vi "generic_PID.vi"(6 "initiation":dbl format="%#_13g", 7 "sensor input":dbl, 8 "setpoint":dbl, 9 "Kd":dbl format="%#_13g", 10 "KI":dbl format="%#_13g", 11 "Kp":dbl format="%#_13g") -> (1 "error":dbl, 2 "PID":dbl)   [LabVIEW 2018]
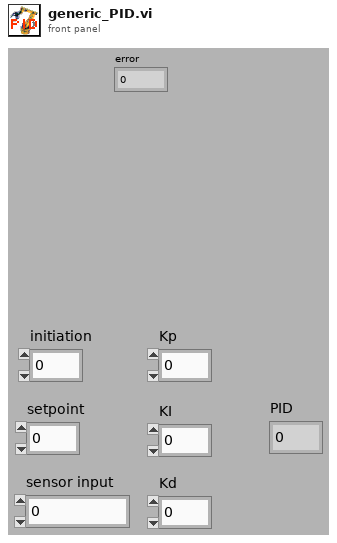
[diagram p1: front panel]
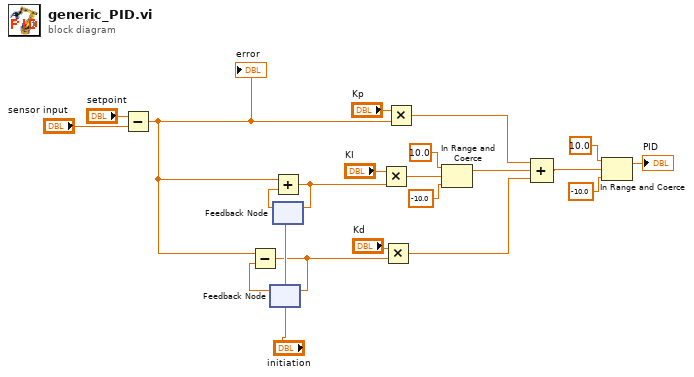
[diagram p0: block diagram]
diagram:
  n1 = Subtract(x="setpoint", y="sensor input") -> (x-y=w17:dbl)
  "error" <- w17
  n2 = feedback #1("initiation") -> (w15:dbl)
  n3 = Subtract(x=w17, y=w15) -> (x-y=w13:dbl)
  n4 = feedback-in #1(w13) -> ()
  n5 = feedback #2("initiation") -> (w16:dbl)
  n6 = Add(x=w17, y=w16) -> (x+y=w14:dbl)
  n7 = feedback-in #2(w14) -> ()
  n8 = Multiply(x="KI", y=w14) -> (x*y=w5:dbl)
  n9 = Multiply(x="Kd", y=w13) -> (x*y=w12:dbl)
  n10 = Multiply(x="Kp", y=w17) -> (x*y=w11:dbl)
  n11 = In Range and Coerce(upper limit=10.0, x=w5, lower limit=-10.0) -> (coerced(x)=w6:dbl)  [unwired: 1 out]
  n12 = Compound Arithmetic op=ADD(w11, w6, w12) -> (w2:dbl)
  n13 = In Range and Coerce(upper limit=10.0, x=w2, lower limit=-10.0) -> (coerced(x)=→"PID":dbl)  [unwired: 1 out]
